vi "lab4_2.vi"() -> ()   [LabVIEW 2021]
panel:
  out "C":dbl(slide) scale=0.0..100.0
  in  "F":dbl(slide) scale=0.0..100.0
  out "F":dbl(slide) scale=0.0..100.0
  in  "C":dbl(slide) scale=0.0..100.0
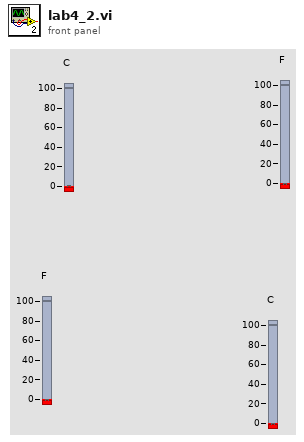
[diagram p1: front panel]
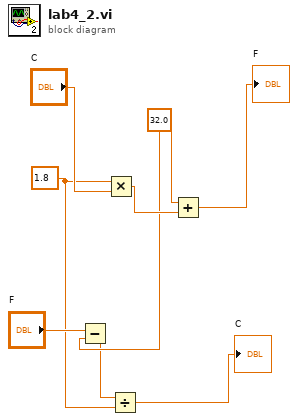
[diagram p0: block diagram]
diagram:
  w4 = 32.0 ("x")
  w2 = 1.8 ("x")
  n1 = Subtract(x="F", y=w4) -> (x-y=w3:dbl)
  n2 = Multiply(x=w2, y="C") -> (x*y=w7:dbl)
  n3 = Divide(x=w3, y=w2) -> (x/y=→"C":dbl)
  n4 = Add(x=w4, y=w7) -> (x+y=→"F":dbl)
